vi "searchForValueParent.vi"(8 "error in (no error)":errorcluster, 9 "nodePath":string, 10 "value":string, 11 "xmlNode in":refnum<class "xmlNode.lvclass">) -> (0 "error out":errorcluster, 2 "Array":string[](array[string]), 3 "xmlNode out":refnum<class "xmlNode.lvclass">)   [LabVIEW 2011, in "Tools.lvlib" / "xml.lvlib" / "xmlNode.lvclass"]
uses:
  xmlNode.lvclass
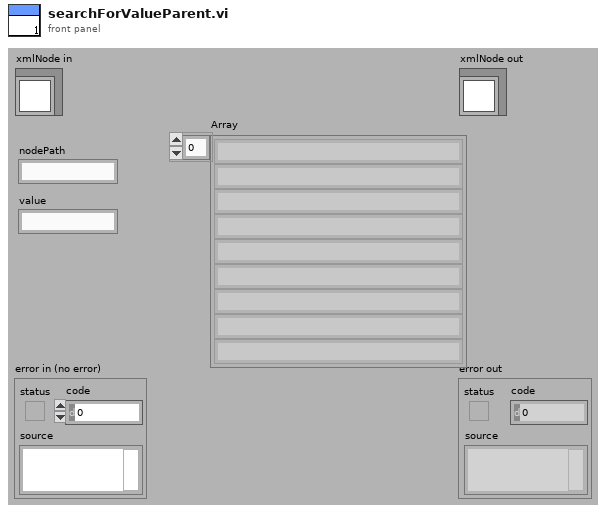
[diagram p1: front panel]
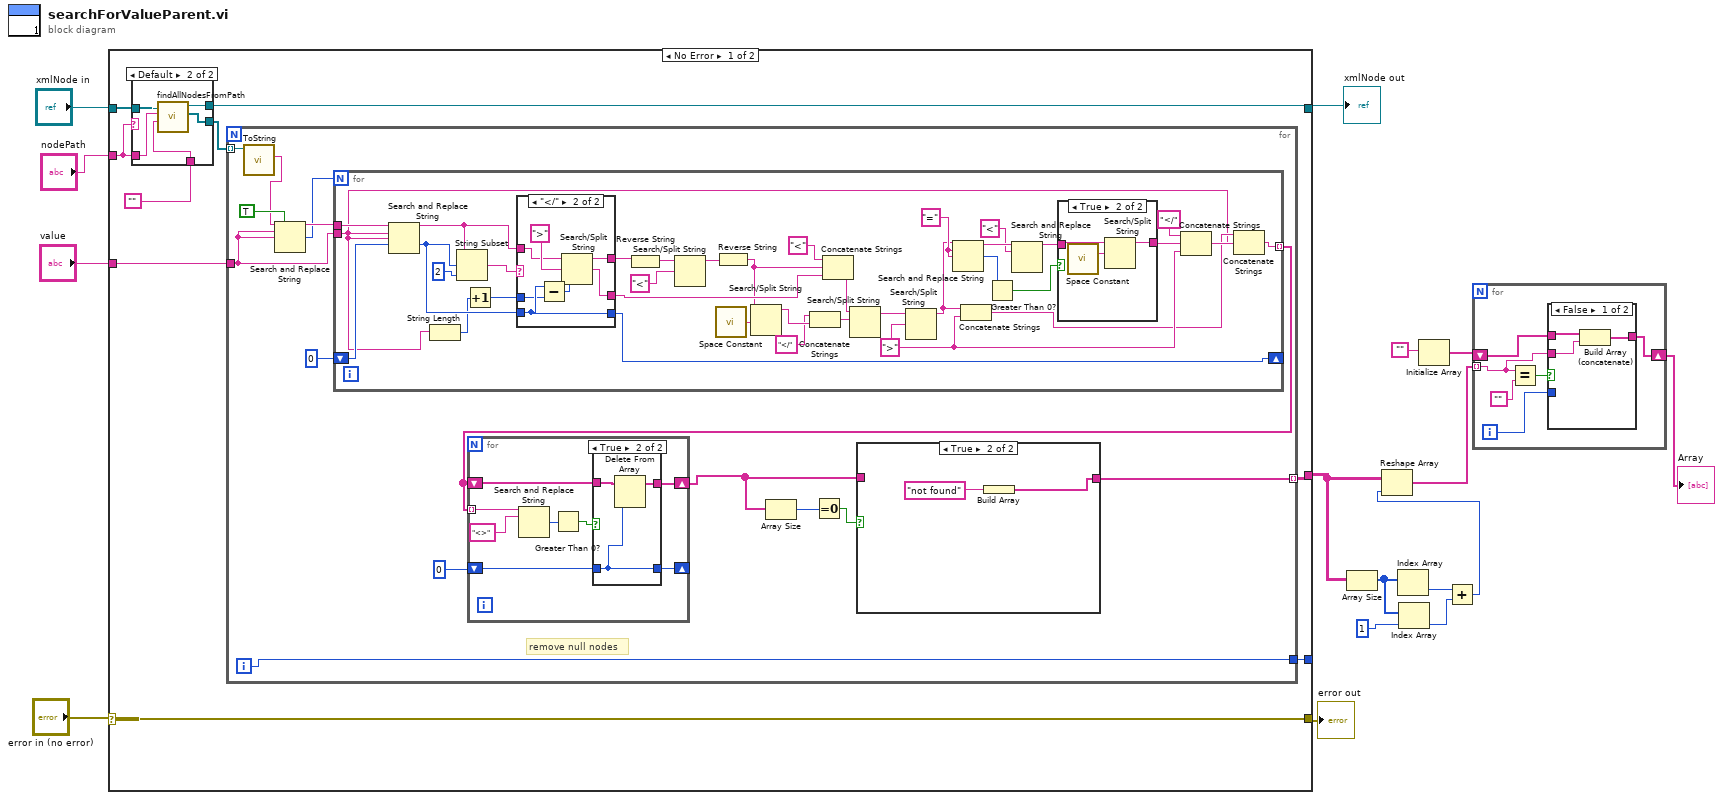
[diagram p0: block diagram]
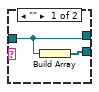
[diagram p3: hidden frame]
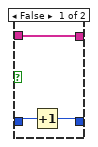
[diagram p5: hidden frame]
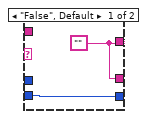
[diagram p7: hidden frame]
diagram:
  n1 = case shown="No Error" "error in (no error)" {
    selector: "error in (no error)" -> [w25 w114]
    tunnel: [w25 w114] -> w15
    tunnel: [w21 w113] -> w13
    tunnel: "xmlNode in" -> [w22 w113]
    tunnel: "value" -> [w24 _]
    tunnel: [w23 _] -> w5
    tunnel: "nodePath" -> [w17 _]
    tunnel: [w19 _] -> _
    frame No Error {
      n2 = case shown="Default" w17 {
        tunnel: w22 -> [w27 w32]
        tunnel: [w27 w31] -> w21
        tunnel: w17 -> [_ w30]
        tunnel: [w26 w29] -> w20
        tunnel: "" -> [_ w28]
        frame "" {
          n3 = Build Array(w27) -> (w26:refnum<class "xmlNode.lvclass">[])
        }
        frame Default {
          n4 = call "findAllNodesFromPath.vi"("searchElement"=w28, "nodePath"=w30, "xmlNode in"=w32) -> ("arrayXmlNodes"=w29:refnum<class "xmlNode.lvclass">[], "xmlNode out"=w31:refnum<class "xmlNode.lvclass">)  [unwired: 6 in, 1 out]
        }
      }
      n5 = for {
        tunnel: w24 -> [w40]
        tunnel: [w36] -> w23 mode=indexing
        tunnel: w20 -> [w34] mode=indexing
        tunnel: [w33] -> w19
        i -> [w33]
        # "remove null nodes"
        n6 = call-dynamic "ToString.vi"("xmlNode in"=w34) -> ("xml"=w39:string)  [unwired: 8 in, 2 out]
        n7 = Search and Replace String(replace all?=TRUE, input string=w39, search string=w40, replace string=w40) -> (result string=w46:string, number of replacements=w44:i32)  [unwired: 4 in, 2 out]
        n8 = for {
          N: w44 -> [_]
          tunnel: w46 -> [w99]
          tunnel: w40 -> [w75]
          shift-right: [w65] -> _
          shift-left: 0 -> [w91]
          tunnel: [w83] -> w42 mode=indexing
          w89 = "="
          w85 = ">"
          n9 = Search and Replace String(input string=w99, search string=w75, replace string=w75, offset=w91) -> (result string=w95:string, offset past replacement=w96:i32)  [unwired: 4 in, 2 out]
          n10 = String Length(string=w75) -> (length=w74:i32)
          n11 = String Subset(string=w95, offset (0)=w96, length (rest)=2) -> (substring=w98:string)
          n12 = Increment(x=w74) -> (x+1=w73:i32)
          n13 = case shown="\"</\"" w98 {
            tunnel: w96 -> [w105 w108]
            tunnel: [w104 w110] -> w93
            tunnel: w95 -> [_ w111]
            tunnel: [w105 w108] -> w65
            tunnel: w73 -> [_ w107]
            tunnel: [w104 w106] -> w72
            frame "False", Default {
              w104 = ""
            }
            frame "</" {
              n14 = Subtract(x=w108, y=w107) -> (x-y=w109:i32)
              n15 = Search/Split String(string=w111, search string/char (-)=">", offset (0)=w109) -> (substring before match=w110:string, match + rest of string=w106:string)  [unwired: 1 out]
            }
          }
          n16 = Reverse String(1:w93) -> (0:w94:string)
          n17 = Search/Split String(string=w94, search string/char (-)="<") -> (substring before match=w92:string)  [unwired: 1 in, 2 out]
          n18 = call <vilib>:"Space Constant.vi"() -> ("String"=w69:string)
          n19 = Reverse String(1:w92) -> (0:w70:string)
          n20 = Search/Split String(string=w70, search string/char (-)=w69) -> (substring before match=w67:string)  [unwired: 1 in, 2 out]
          n21 = Concatenate Strings("</", w67) -> (w68:string)
          n22 = Concatenate Strings("<", w70, w72) -> (w71:string)
          n23 = Search/Split String(string=w71, search string/char (-)=w68) -> (substring before match=w64:string)  [unwired: 1 in, 2 out]
          n24 = Search/Split String(string=w64, search string/char (-)=w85) -> (substring before match=w81:string)  [unwired: 1 in, 2 out]
          n25 = Search and Replace String(input string=w81, search string=w89, replace string=w89) -> (result string=w77:string, number of replacements=w88:i32)  [unwired: 5 in, 2 out]
          n26 = Concatenate Strings(w81, w85) -> (w82:string)
          n27 = Greater Than 0?(x=w88) -> (x > 0?=w87:bool)
          n28 = Search and Replace String(input string=w77, search string="<") -> (result string=w78:string)  [unwired: 6 in, 3 out]
          n29 = case shown="True" w87 {
            tunnel: w78 -> [w100 w103]
            tunnel: [w100 w101] -> w86
            frame False {
            }
            frame True {
              n30 = call <vilib>:"Space Constant.vi"() -> ("String"=w102:string)
              n31 = Search/Split String(string=w103, search string/char (-)=w102) -> (substring before match=w101:string)  [unwired: 1 in, 2 out]
            }
          }
          n32 = Concatenate Strings("</", w86, w85) -> (w84:string)
          n33 = Concatenate Strings(w82, w75, w84) -> (w83:string)
        }
        n34 = for {
          tunnel: w42 -> [w57] mode=indexing
          shift-right: [w52] -> w37
          shift-left: w42 -> [w53]
          shift-right: [w50] -> _
          shift-left: 0 -> [w51]
          n35 = Search and Replace String(input string=w57, search string="<>") -> (number of replacements=w55:i32)  [unwired: 6 in, 3 out]
          n36 = Greater Than 0?(x=w55) -> (x > 0?=w54:bool)
          n37 = case shown="True" w54 {
            tunnel: w53 -> [w60 w63]
            tunnel: [w60 w62] -> w52
            tunnel: w51 -> [w59 w61]
            tunnel: [w58 w61] -> w50
            frame False {
              n38 = Increment(x=w59) -> (x+1=w58:i32)
            }
            frame True {
              n39 = Delete From Array(array=w63, index=w61) -> (array with subset deleted=w62:string[])  [unwired: 1 in, 1 out]
            }
          }
        }
        n40 = Array Size(array=w37) -> (size(s)=w38:i32)
        n41 = Equal To 0?(x=w38) -> (x = 0?=w35:bool)
        n42 = case shown="True" w35 {
          tunnel: [w47 w48] -> w36
          tunnel: w37 -> [w47 _]
          frame False {
          }
          frame True {
            n43 = Build Array("not found") -> (w48:string[])
          }
        }
      }
    }
    frame Error {
    }
  }
  "error out" <- w15
  "xmlNode out" <- w13
  n44 = Array Size(array=w5) -> (size(s)=w10:i32[])
  n45 = Index Array(array=w10) -> (element=w8:i32)  [unwired: 1 in]
  n46 = Index Array(array=w10, index=1) -> (element=w7:i32)
  n47 = Initialize Array("") -> (w2:string[])  [unwired: 1 in]
  n48 = Add(x=w8, y=w7) -> (x+y=w6:i32)
  n49 = Reshape Array(w5, w6) -> (w4:string[])
  n50 = for {
    tunnel: w4 -> [w115] mode=indexing
    shift-right: [w116] -> w3
    shift-left: w2 -> [w118]
    i -> [w117]
    n51 = Equal?(x=w115, y="") -> (x = y?=w119:bool)
    n52 = case shown="False" w119 {
      tunnel: w118 -> [w123 w124]
      tunnel: w117 -> [_ _]
      tunnel: [w121 w124] -> w116
      tunnel: w115 -> [w122 _]
      frame False {
        n53 = Build Array (concatenate)(w123, w122) -> (w121:string[])
      }
      frame True {
      }
    }
  }
  "Array" <- w3
